vi "Send Set Minimum Panel Size.vi"(7 "Message Priority (Normal)":T2=enum."Normal", 8 "error in (no error)":errorcluster, 10 "Minimum Size":T1, 11 "Message Enqueuer":refnum<class "Message Enqueuer.lvclass">) -> (0 "error out":errorcluster, 3 "Message Enqueuer out":refnum<class "Message Enqueuer.lvclass">)   [LabVIEW 2017, in "IViewable.lvlib" / "Set Minimum Panel Size Msg.lvclass"]
doc: "This VI sends the message to an actor."
uses:
  Set Minimum Panel Size Msg.lvclass
  <vilib>/ActorFramework/Message Enqueuer/Message Enqueuer.lvclass
  <vilib>/ActorFramework/Message Enqueuer/Message Priority.ctl
  <vilib>/Utility/miscctls.llb/LVPointTypeDef.ctl
  C:/Program Files (x86)/National Instruments/LabVIEW 2017/vi.lib/ActorFramework/Message/Message.lvclass
  Set Minimum Panel Size Msg.lvclass/Set Minimum Panel Size Msg.ctl
  <vilib>/ActorFramework/Message Enqueuer/Message Enqueuer.lvclass/Message Enqueuer.ctl
  <vilib>/ActorFramework/Message Priority Queue/Priority Enqueue.vi
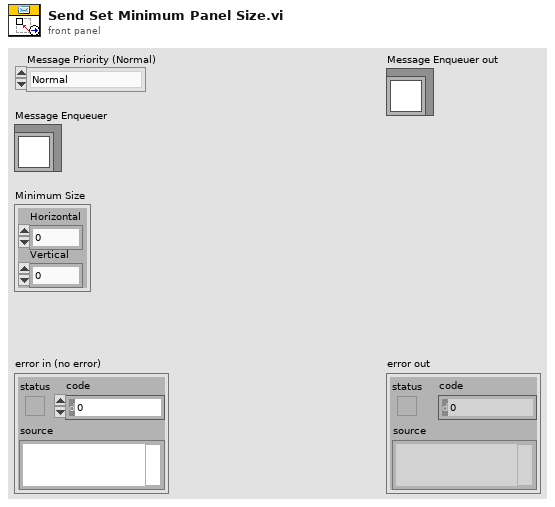
[diagram p1: front panel]
types:
  T1 = typedef "LVPointTypeDef.ctl" = cluster{"Horizontal":i16, "Vertical":i16}
  T2 = typedef "Actor Framework.lvlib/Message Enqueuer.lvclass/Message Priority.ctl" = enum16{"Low", "Normal", "High"}
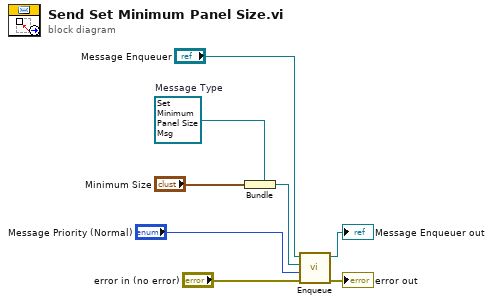
[diagram p0: block diagram]
diagram:
  w2 = refnum<class "Set Minimum Panel Size Msg.lvclass"> refnum  # Message Type
  n1 = Bundle(cluster=w2, "Minimum Size") -> (w3:refnum<class "Set Minimum Panel Size Msg.lvclass">)
  n2 = call <vilib>:"Enqueue.vi"("error in (no error)"="error in (no error)", "Message Priority (Normal)"="Message Priority (Normal)", "Message"=w3, "Message Enqueuer in"="Message Enqueuer") -> ("error out"=→"error out":errorcluster, "Message Enqueuer out"=→"Message Enqueuer out":refnum<class "Message Enqueuer.lvclass">)  [unwired: 6 in]
